vi "Put Control on Cursor.vi"(8 "error in (no error)":errorcluster, 10 "Control":string, 11 "Editor in":refnum<class "Editor.lvclass">) -> (0 "error out":errorcluster, 3 "Editor out":refnum<class "Editor.lvclass">)   [LabVIEW 2020, in "VolatusGUIEditor.lvlib" / "Editor.lvclass"]
uses:
  Editor.lvclass
  Editor.lvclass/Editor.ctl
  Control List/Control List.lvclass
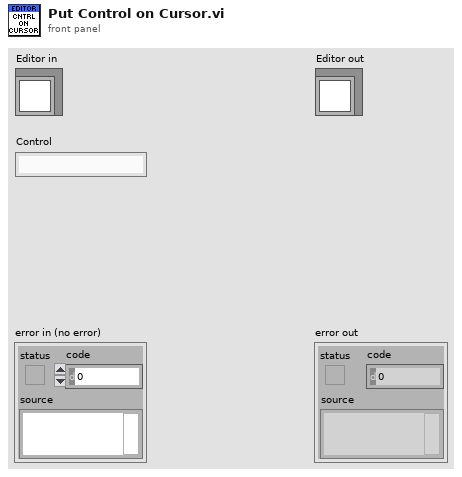
[diagram p1: front panel]
types:
  T1 = typedef "VolatusGUIEditor.lvlib/Control Info.ctl" = cluster{"Description":string, "Hierarchy":string[], "Image":T2, "Element Type":string, "Path":path}
  T2 = typedef "imagedata.ctl" = cluster{"image type":i32, "image depth":i32, "image":u8[], "mask":u8[], "colors":u32[], "Rectangle":cluster{"left":i16, "top":i16, "right":i16, "bottom":i16}}
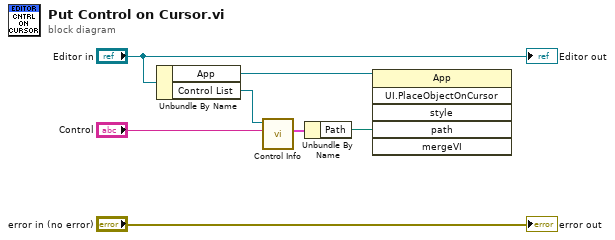
[diagram p0: block diagram]
diagram:
  n1 = Unbundle By Name("Editor in") -> ("App"=w1:refnum<vi>, "Control List"=w5:refnum<class "Control List.lvclass">)
  n2 = call "Control Info.vi"("Control Type"="Control", "Control List in"=w5) -> ("Control Info"=w3:T1)  [unwired: 7 in, 2 out]
  n3 = Unbundle By Name(w3) -> ("Path"=w2:path)
  n4 = invoke class="App" method="UI.PlaceObjectOnCursor"(reference=w1, "path"=w2) -> ()  [unwired: 4 in, 6 out]
  "error out" <- "error in (no error)"
  "Editor out" <- "Editor in"
